vi "controlVisibility4Ch.vi"(7 "device type [AB1004]":T2=1004 items=["any"=0, "AB1002"=1002, "AB1004"=1004, "AB1502"=1502, "AB1504"=1504, "AB2002"=2002, "AB2004"=2004, "AB2502"=2502, "AB2504"=2504], 9 "ref controls":T1, 10 "connection state":T3) -> ()   [LabVIEW 2015]
doc: "Sets the visibility of control inputs on front panel at \"Tausand AB1000 Acquisition Example.vi\", depending on the current connection state.\nSets the increment and minimum of digital controls."
uses:
  <instrlib>/Tausand AB1000/Examples/sub vi/connectionState.ctl
  <instrlib>/Tausand AB1000/Public/Controls/deviceTypeRing.ctl
  <instrlib>/Tausand AB1000/Public/Controls/settings2ch.ctl
  <instrlib>/Tausand AB1000/Public/Controls/settings4ch.ctl
  <instrlib>/Tausand AB1000/Public/Controls/configMultipleCoincRing.ctl
  <instrlib>/Tausand AB1000/Tausand AB1000.lvlib
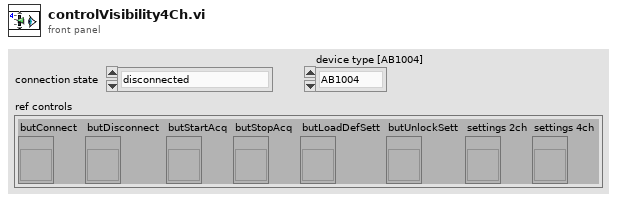
[diagram p1: front panel]
types:
  T1 = cluster{"butConnect":refnum<vi>, "butDisconnect":refnum<vi>, "butStartAcq":refnum<vi>, "butStopAcq":refnum<vi>, "butLoadDefSett":refnum<vi>, "butUnlockSett":refnum<vi>, "settings 2ch":refnum<vi>, "settings 4ch":refnum<vi>}
  T2 = typedef "Tausand AB1000.lvlib/deviceTypeRing.ctl" = u16
  T3 = typedef "connectionState.ctl" = enum16{"disconnected", "connected", "acquiring data", "connection error", "acquisition error"}
  T4 = enum8{"Enabled", "Disabled", "Disabled and Grayed Out"}
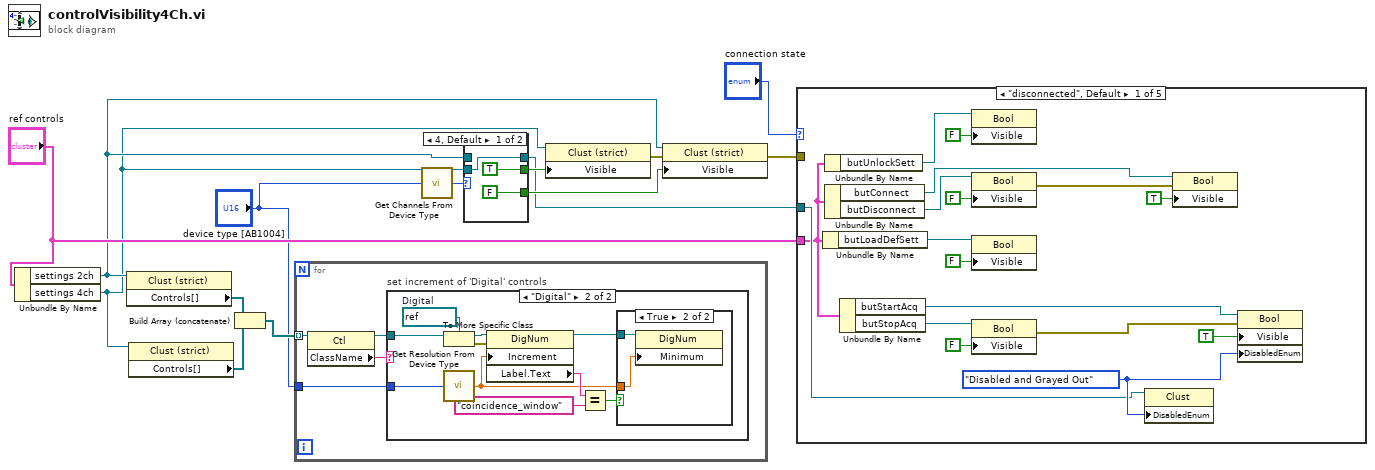
[diagram p0: block diagram]
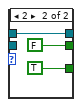
[diagram p4: hidden frame]
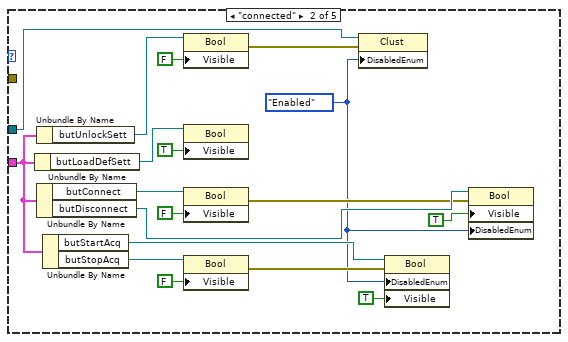
[diagram p5: hidden frame]
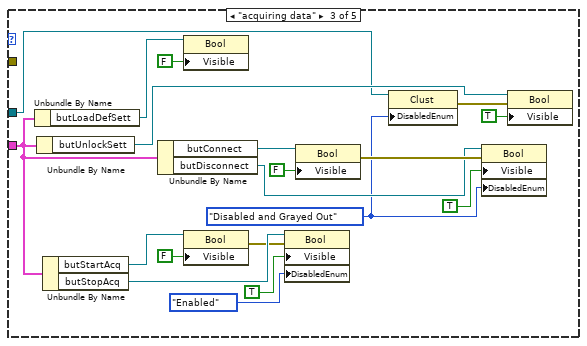
[diagram p6: hidden frame]
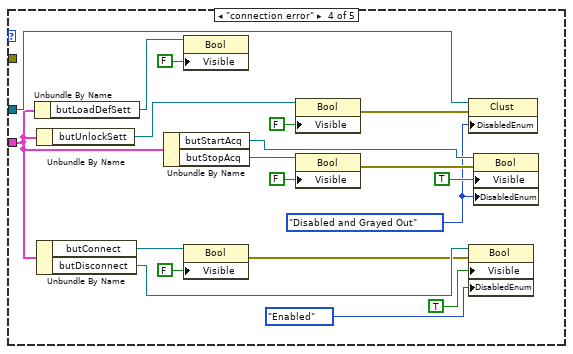
[diagram p7: hidden frame]
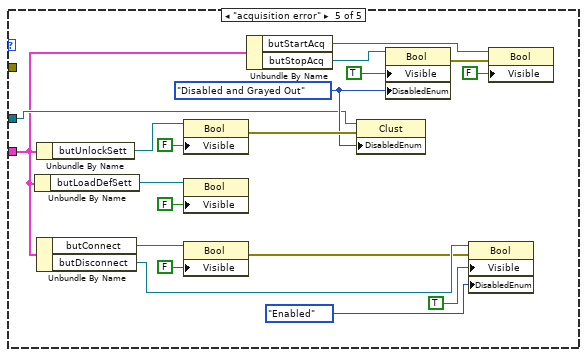
[diagram p8: hidden frame]
diagram:
  n1 = Unbundle By Name("ref controls") -> ("settings 2ch"=w7:refnum<vi>, "settings 4ch"=w6:refnum<vi>)
  n2 = property class="Clust (strict)"(reference=w7) -> ("Controls[]"=w5:refnum<vi>[])  [unwired: 1 in, 2 out]
  n3 = property class="Clust (strict)"(reference=w6) -> ("Controls[]"=w4:refnum<vi>[])  [unwired: 1 in, 2 out]
  n4 = Build Array (concatenate)(w5, w4) -> (w3:refnum<vi>[])
  n5 = for {
    tunnel: w3 -> [w15] mode=indexing
    tunnel: "device type [AB1004]" -> [w16]
    n6 = property class="Ctl"(reference=w15) -> (reference out=w18:refnum<vi>, "ClassName"=w17:string)  [unwired: 1 in, 1 out]
    n7 = case "set increment of 'Digital' controls" shown="\"Digital\"" w17 {
      tunnel: w18 -> [_ w27]
      tunnel: w16 -> [_ w24]
      frame "False", Default {
      }
      frame "Digital" {
        w28 = refnum<vi> refnum  # Digital
        n8 = To More Specific Class(target class=w28, reference=w27) -> (specific class reference=w25:refnum<vi>, error out=w26:errorcluster)  [unwired: 1 in]
        n9 = call <instrlib>:"Get Resolution From Device Type.vi"("device type"=w24) -> ("resolution [ns]"=w21:dbl)  [unwired: 4 in]
        n10 = property class="DigNum"(reference=w25, error in=w26, "Increment"=w21) -> (reference out=w20:refnum<vi>, "Label.Text"=w23:string)  [unwired: 1 out]
        n11 = Equal?(x=w23, y="coincidence_window") -> (x = y?=w19:bool)
        n12 = case shown="True" w19 {
          tunnel: w21 -> [_ w30]
          tunnel: w20 -> [_ w29]
          frame False {
          }
          frame True {
            n13 = property class="DigNum"(reference=w29, "Minimum"=w30) -> ()  [unwired: 1 in, 2 out]
          }
        }
      }
    }
  }
  n14 = call <instrlib>:"Get Channels From Device Type.vi"("device type"="device type [AB1004]") -> ("channels"=w1:i32)  [unwired: 4 in]
  n15 = case shown="4, Default" w1 {
    tunnel: [FALSE TRUE] -> w13
    tunnel: [TRUE FALSE] -> w12
    tunnel: [w31 w34] -> w9
    tunnel: w6 -> [w31 _]
    tunnel: w7 -> [_ w34]
    frame 4, Default {
    }
    frame 2 {
    }
  }
  n16 = property class="Clust (strict)"(reference=w6, "Visible"=w12) -> (error out=w11:errorcluster)  [unwired: 1 in, 1 out]
  n17 = property class="Clust (strict)"(reference=w7, error in=w11, "Visible"=w13) -> (error out=w10:errorcluster)  [unwired: 1 out]
  n18 = case shown="\"disconnected\", Default" "connection state" {
    tunnel: "ref controls" -> [w37 w54 w74 w91 w110]
    tunnel: w10 -> [_ _ _ _ _]
    tunnel: w9 -> [w40 w57 w75 w94 w113]
    frame "disconnected", Default {
      w46 = T4."Disabled and Grayed Out" ("Disabled")
      n19 = Unbundle By Name(w37) -> ("butLoadDefSett"=w39:refnum<vi>)
      n20 = Unbundle By Name(w37) -> ("butUnlockSett"=w48:refnum<vi>)
      n21 = Unbundle By Name(w37) -> ("butConnect"=w44:refnum<vi>, "butDisconnect"=w43:refnum<vi>)
      n22 = Unbundle By Name(w37) -> ("butStartAcq"=w42:refnum<vi>, "butStopAcq"=w41:refnum<vi>)
      n23 = property class="Bool"(reference=w48, "Visible"=FALSE) -> ()  [unwired: 1 in, 2 out]
      n24 = property class="Bool"(reference=w43, "Visible"=FALSE) -> (error out=w45:errorcluster)  [unwired: 1 in, 1 out]
      n25 = property class="Bool"(reference=w39, "Visible"=FALSE) -> ()  [unwired: 1 in, 2 out]
      n26 = property class="Bool"(reference=w41, "Visible"=FALSE) -> (error out=w47:errorcluster)  [unwired: 1 in, 1 out]
      n27 = property class="Clust"(reference=w40, "DisabledEnum"=w46) -> ()  [unwired: 1 in, 2 out]
      n28 = property class="Bool"(reference=w44, error in=w45, "Visible"=TRUE) -> ()  [unwired: 2 out]
      n29 = property class="Bool"(reference=w42, error in=w47, "Visible"=TRUE, "DisabledEnum"=w46) -> ()  [unwired: 2 out]
    }
    frame "connected" {
      w58 = T4."Enabled" ("Disabled")
      n30 = Unbundle By Name(w54) -> ("butLoadDefSett"=w56:refnum<vi>)
      n31 = Unbundle By Name(w54) -> ("butUnlockSett"=w60:refnum<vi>)
      n32 = Unbundle By Name(w54) -> ("butConnect"=w71:refnum<vi>, "butDisconnect"=w67:refnum<vi>)
      n33 = Unbundle By Name(w54) -> ("butStartAcq"=w68:refnum<vi>, "butStopAcq"=w65:refnum<vi>)
      n34 = property class="Bool"(reference=w60, "Visible"=FALSE) -> (error out=w59:errorcluster)  [unwired: 1 in, 1 out]
      n35 = property class="Bool"(reference=w56, "Visible"=TRUE) -> ()  [unwired: 1 in, 2 out]
      n36 = property class="Bool"(reference=w71, "Visible"=FALSE) -> (error out=w66:errorcluster)  [unwired: 1 in, 1 out]
      n37 = property class="Bool"(reference=w65, "Visible"=FALSE) -> (error out=w62:errorcluster)  [unwired: 1 in, 1 out]
      n38 = property class="Clust"(reference=w57, error in=w59, "DisabledEnum"=w58) -> ()  [unwired: 2 out]
      n39 = property class="Bool"(reference=w68, error in=w62, "DisabledEnum"=w58, "Visible"=TRUE) -> ()  [unwired: 2 out]
      n40 = property class="Bool"(reference=w67, error in=w66, "Visible"=TRUE, "DisabledEnum"=w58) -> ()  [unwired: 2 out]
    }
    frame "acquiring data" {
      w79 = T4."Disabled and Grayed Out" ("Disabled")
      n41 = Unbundle By Name(w74) -> ("butLoadDefSett"=w72:refnum<vi>)
      n42 = Unbundle By Name(w74) -> ("butUnlockSett"=w77:refnum<vi>)
      n43 = Unbundle By Name(w74) -> ("butStartAcq"=w90:refnum<vi>, "butStopAcq"=w89:refnum<vi>)
      n44 = Unbundle By Name(w74) -> ("butConnect"=w81:refnum<vi>, "butDisconnect"=w80:refnum<vi>)
      n45 = property class="Bool"(reference=w72, "Visible"=FALSE) -> ()  [unwired: 1 in, 2 out]
      n46 = property class="Bool"(reference=w90, "Visible"=FALSE) -> (error out=w86:errorcluster)  [unwired: 1 in, 1 out]
      n47 = property class="Bool"(reference=w89, error in=w86, "Visible"=TRUE, "DisabledEnum"=T4."Enabled" ("Disabled")) -> ()  [unwired: 2 out]
      n48 = property class="Bool"(reference=w81, "Visible"=FALSE) -> (error out=w82:errorcluster)  [unwired: 1 in, 1 out]
      n49 = property class="Clust"(reference=w75, "DisabledEnum"=w79) -> (error out=w76:errorcluster)  [unwired: 1 in, 1 out]
      n50 = property class="Bool"(reference=w80, error in=w82, "Visible"=TRUE, "DisabledEnum"=w79) -> ()  [unwired: 2 out]
      n51 = property class="Bool"(reference=w77, error in=w76, "Visible"=TRUE) -> ()  [unwired: 2 out]
    }
    frame "connection error" {
      w95 = T4."Disabled and Grayed Out" ("Disabled")
      n52 = Unbundle By Name(w91) -> ("butLoadDefSett"=w93:refnum<vi>)
      n53 = Unbundle By Name(w91) -> ("butUnlockSett"=w99:refnum<vi>)
      n54 = Unbundle By Name(w91) -> ("butConnect"=w109:refnum<vi>, "butDisconnect"=w105:refnum<vi>)
      n55 = Unbundle By Name(w91) -> ("butStartAcq"=w106:refnum<vi>, "butStopAcq"=w103:refnum<vi>)
      n56 = property class="Bool"(reference=w93, "Visible"=FALSE) -> ()  [unwired: 1 in, 2 out]
      n57 = property class="Bool"(reference=w109, "Visible"=FALSE) -> (error out=w104:errorcluster)  [unwired: 1 in, 1 out]
      n58 = property class="Bool"(reference=w99, "Visible"=FALSE) -> (error out=w98:errorcluster)  [unwired: 1 in, 1 out]
      n59 = property class="Bool"(reference=w103, "Visible"=FALSE) -> (error out=w101:errorcluster)  [unwired: 1 in, 1 out]
      n60 = property class="Clust"(reference=w94, error in=w98, "DisabledEnum"=w95) -> ()  [unwired: 2 out]
      n61 = property class="Bool"(reference=w105, error in=w104, "Visible"=TRUE, "DisabledEnum"=T4."Enabled" ("Disabled")) -> ()  [unwired: 2 out]
      n62 = property class="Bool"(reference=w106, error in=w101, "Visible"=TRUE, "DisabledEnum"=w95) -> ()  [unwired: 2 out]
    }
    frame "acquisition error" {
      w114 = T4."Disabled and Grayed Out" ("Disabled")
      n63 = Unbundle By Name(w110) -> ("butLoadDefSett"=w112:refnum<vi>)
      n64 = Unbundle By Name(w110) -> ("butUnlockSett"=w118:refnum<vi>)
      n65 = Unbundle By Name(w110) -> ("butConnect"=w128:refnum<vi>, "butDisconnect"=w124:refnum<vi>)
      n66 = property class="Bool"(reference=w118, "Visible"=FALSE) -> (error out=w117:errorcluster)  [unwired: 1 in, 1 out]
      n67 = property class="Bool"(reference=w112, "Visible"=FALSE) -> ()  [unwired: 1 in, 2 out]
      n68 = property class="Bool"(reference=w128, "Visible"=FALSE) -> (error out=w123:errorcluster)  [unwired: 1 in, 1 out]
      n69 = Unbundle By Name(w110) -> ("butStartAcq"=w125:refnum<vi>, "butStopAcq"=w122:refnum<vi>)
      n70 = property class="Clust"(reference=w113, error in=w117, "DisabledEnum"=w114) -> ()  [unwired: 2 out]
      n71 = property class="Bool"(reference=w122, "Visible"=TRUE, "DisabledEnum"=w114) -> (error out=w120:errorcluster)  [unwired: 1 in, 1 out]
      n72 = property class="Bool"(reference=w124, error in=w123, "Visible"=TRUE, "DisabledEnum"=T4."Enabled" ("Disabled")) -> ()  [unwired: 2 out]
      n73 = property class="Bool"(reference=w125, error in=w120, "Visible"=FALSE) -> ()  [unwired: 2 out]
    }
  }
